vi "Find Maximum and Minimum Indexes.vi"(10 "broken streaks":u8[](array[numeric]), 11 "map":i8[](array[numeric])) -> (2 "minimum indexes":u8[](array[numeric]), 3 "maximum indexes":u8[](array[numeric]))   [LabVIEW 2022 SP3]
uses:
  Broken Springs Block Math.vi
  Increment Indexes.vi
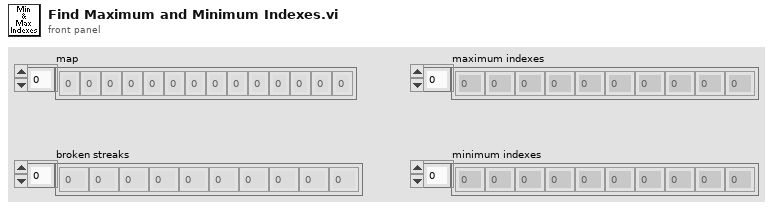
[diagram p1: front panel]
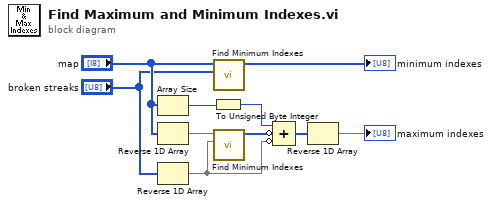
[diagram p0: block diagram]
diagram:
  n1 = Array Size(array="map") -> (size(s)=w10:i32)
  n2 = Reverse 1D Array(array="map") -> (reversed array=w5:i8[])
  n3 = Reverse 1D Array(array="broken streaks") -> (reversed array=w6:u8[])
  n4 = To Unsigned Byte Integer(number=w10) -> (unsigned 8bit integer=w8:u8)
  n5 = call "Find Minimum Indexes.vi"("broken streaks"="broken streaks", "map"="map") -> ("minimum indexes"=→"minimum indexes":u8[])  [unwired: 9 in]
  n6 = call "Find Minimum Indexes.vi"("broken streaks"=w6, "map"=w5) -> ("minimum indexes"=w7:u8[])  [unwired: 9 in]
  n7 = Compound Arithmetic op=ADD(w8, invert w7, invert w6) -> (w1:u8[])
  n8 = Reverse 1D Array(array=w1) -> (reversed array=→"maximum indexes":u8[])
